vi "Server INFO.vi"() -> ()   [LabVIEW 2019, in "Redis Client Examples.lvlib"]
uses:
  Redis Client Examples.lvlib
  Redis Client for LabVIEW/Redis TCP Client/Redis TCP Client.lvclass
  C:/Users/Nicholas Folse/Documents/workspace/github-tauterra.llc/Redis Client for LabVIEW/Redis Client for LabVIEW/Redis Client/Redis Client.lvclass
  Redis Client for LabVIEW/Redis Client/Redis Client.lvclass
panel:
  in  "section":string
  out "INFO":string
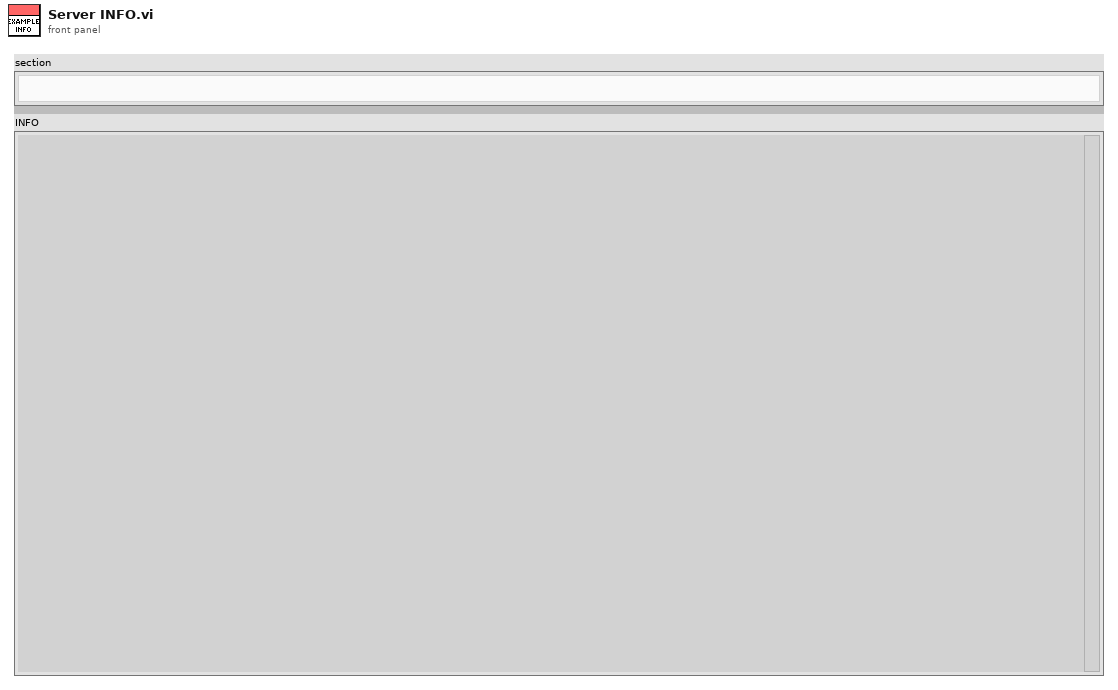
[diagram p1: front panel]
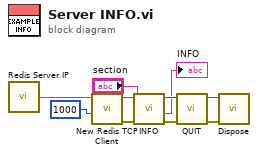
[diagram p0: block diagram]
diagram:
  n1 = call "Redis Server IP.vi"() -> ("server IP"=w10:string)
  n2 = call "New Redis TCP Client.vi"("timeout ms (25000)"=1000, "address"=w10) -> ("error out"=w7:errorcluster, "Redis TCP Client out"=w8:refnum<class "Redis TCP Client.lvclass">)  [unwired: 8 in]
  n3 = call "INFO.vi"("error in (no error)"=w7, "section"="section", "Redis Client in"=w8) -> ("error out"=w6:errorcluster, "info"=→"INFO":string, "Redis Client out"=w5:refnum<class "Redis TCP Client.lvclass">)  [unwired: 6 in]
  n4 = call "QUIT.vi"("error in (no error)"=w6, "Redis Client in"=w5) -> ("error out"=w3:errorcluster, "Redis Client out"=w4:refnum<class "Redis TCP Client.lvclass">)  [unwired: 8 in]
  n5 = call-dynamic "Dispose.vi"("error in (no error)"=w3, "Redis TCP Client in"=w4) -> ()  [unwired: 9 in, 1 out]
